vi "Test Case - When Not Constructed - Returns Default Value.vi"() -> ()   [LabVIEW 2017, in "Test Result.Tests.lvlib"]
uses:
  Test Result.Tests.lvlib
  Test Result/Test Result.lvclass
  Test Result/Test Result.lvclass/Test Result.ctl
  Test Case/Test Case.lvclass
  Test Result/Get Test Case.vi
  <vilib>/PNR/Transparent Assertions/Transparent Assertions/Transparent Assertions.lvlib
panel:
  out "error out":errorcluster
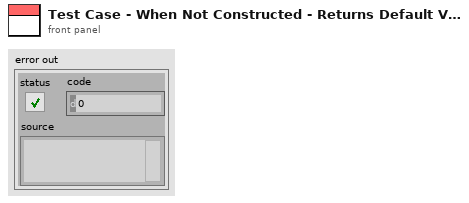
[diagram p1: front panel]
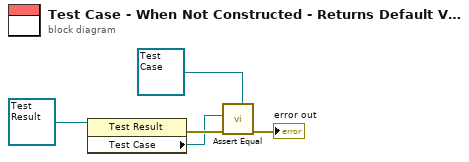
[diagram p0: block diagram]
diagram:
  n1 = property class="Test Result"(reference=refnum<class "Test Result.lvclass"> refnum ("Test Result")) -> (error out=w4:errorcluster, "Test Case"=w3:refnum<class "Test Case.lvclass">)  [unwired: 1 in, 1 out]
  n2 = call <vilib>:"Assert Equal.vi"("Expected"=refnum<class "Test Case.lvclass"> refnum ("Test Case"), "error in (no error)"=w4, "Actual"=w3) -> ("error out"=→"error out":errorcluster)  [unwired: 8 in]
